vi "XIPIN_DDR4_SDRAM_(MIG)_1_1.vi"   [LabVIEW 2017]
doc: "DDR4 Interface Generator for Ultrascale Architecture\n------------------------------------\n<b>Need License</b> : No\n<b>Interface</b> : AXI4"
uses:
  <vilib>/rvi/XilinxIP/XIPIN_XNode/niFpgaXIPIN.xnode
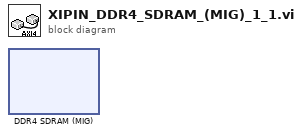
[diagram p0: block diagram]
diagram:
  n1 = xnode ("DDR4 SDRAM (MIG)")() -> ()
